vi "AFT Filter Signal and Update Coefficients (Complex, Waveform).vi"(6 "step size":dbl=-1.0, 7 "reset? (F)":bool, 8 "error in (no error)":errorcluster, 9 "d(n)":waveform(cdb)={"t0"=timestamp(0 s since 1904-01-01), "dt"=0.0, "Y"=[]}, 10 "x(n)":waveform(cdb)={"t0"=timestamp(0 s since 1904-01-01), "dt"=0.0, "Y"=[]}, 11 "adaptive filter in":refnum<k20>) -> (0 "error out":errorcluster, 1 "e(n)":waveform(cdb), 2 "y(n)":waveform(cdb), 3 "adaptive filter out":refnum<k20>)   [LabVIEW 2017, in "NI_AdaptiveFilter.lvlib"]
doc: "Filters an input signal with an adaptive filter and updates the coefficients of the adaptive filter iteratively. You must use the least mean squares (LMS) or recursive least squares (RLS) algorithms to create the adaptive filter. Wire data to the <B>x(n)</B> and <B>d(n)</B> inputs to determine the polymorphic instance to use or manually select the instance. The data type of the adaptive filter that you wire to the <B>adaptive filter in</B> input must match the instance of the AFT Filter Signal and Update Coefficients VI."
uses:
  <vilib>/addons/Adaptive Filters/NI_AdaptiveFilter.lvlib
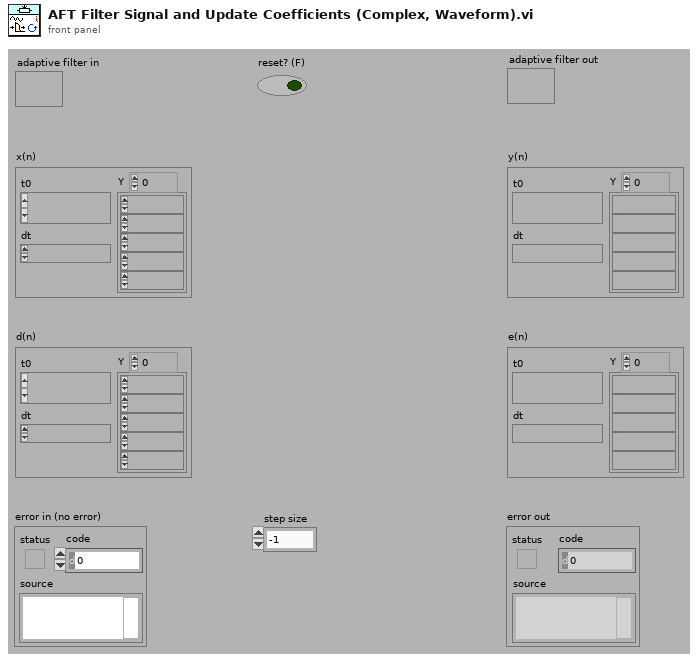
[diagram p1: front panel]
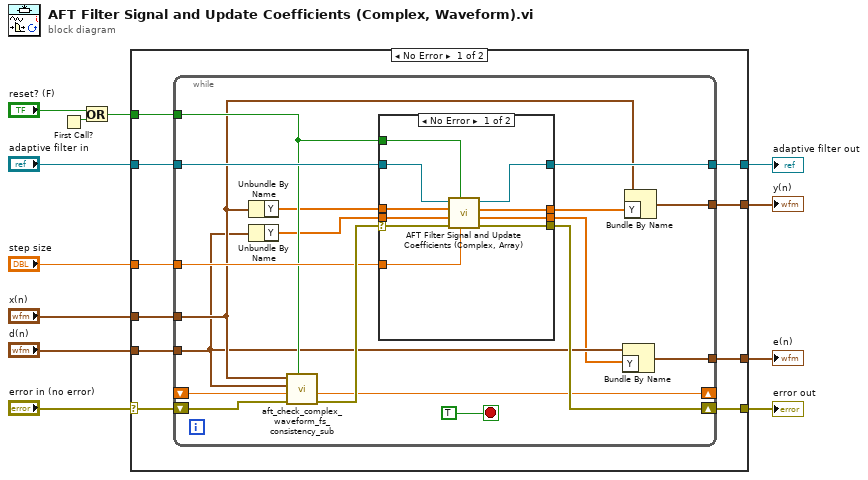
[diagram p0: block diagram]
diagram:
  n1 = First Call?() -> (First Call?: T/F=w5:bool)
  n2 = Or(x="reset? (F)", y=w5) -> (x .or. y?=w4:bool)
  n3 = case shown="No Error" "error in (no error)" {
    selector: "error in (no error)" -> [w20 w53]
    tunnel: "x(n)" -> [w22 _]
    tunnel: "d(n)" -> [w21 _]
    tunnel: "adaptive filter in" -> [w19 w54]
    tunnel: [w18 w54] -> w2
    tunnel: "step size" -> [w17 _]
    tunnel: w4 -> [w16 _]
    tunnel: [w15 w53] -> w8
    tunnel: [w14 _] -> w7
    tunnel: [w13 _] -> w6
    frame No Error {
      n4 = while {
        tunnel: w22 -> [w28]
        tunnel: w21 -> [w27]
        shift-right: [w23] -> _
        shift-left: _ -> [w39]
        shift-right: [w34] -> w15
        shift-left: w20 -> [w38]
        tunnel: w19 -> [w36]
        tunnel: [w35] -> w18
        tunnel: w17 -> [w33]
        tunnel: w16 -> [w32]
        tunnel: [w25] -> w14
        tunnel: [w24] -> w13
        stop <- TRUE stop-if-true
        n5 = Unbundle By Name(w28) -> ("Y"=w31:cdb[])
        n6 = Unbundle By Name(w27) -> ("Y"=w30:cdb[])
        n7 = call <vilib>:"aft_check_complex_waveform_fs_consistency_sub.vi"("init"=w32, "error in (no error)"=w38, "dt in"=w39, "signal in 2"=w27, "signal in 1"=w28) -> ("error out"=w37:errorcluster, "dt out"=w23:dbl)  [unwired: 5 out]
        n8 = case shown="No Error" w37 {
          selector: w37 -> [w50 w51]
          tunnel: w36 -> [w43 w52]
          tunnel: [w42 w52] -> w35
          tunnel: [w49 w51] -> w34
          tunnel: w33 -> [w48 _]
          tunnel: w32 -> [w41 _]
          tunnel: w31 -> [w47 _]
          tunnel: w30 -> [w46 _]
          tunnel: [w45 _] -> w29
          tunnel: [w44 _] -> w26
          frame No Error {
            n9 = call <vilib>:"AFT Filter Signal and Update Coefficients (Complex, Array).vi"("step size"=w48, "reset? (F)"=w41, "error in (no error)"=w50, "d(n)"=w46, "x(n)"=w47, "adaptive filter in"=w43) -> ("error out"=w49:errorcluster, "e(n)"=w44:cdb[], "y(n)"=w45:cdb[], "adaptive filter out"=w42:refnum<k20>)  [unwired: 2 out]
          }
          frame Error {
          }
        }
        n10 = Bundle By Name(cluster=w27, "Y"=w26) -> (w25:waveform(cdb))
        n11 = Bundle By Name(cluster=w28, "Y"=w29) -> (w24:waveform(cdb))
      }
    }
    frame Error {
    }
  }
  "error out" <- w8
  "y(n)" <- w6
  "e(n)" <- w7
  "adaptive filter out" <- w2
